vi "Read Photometric Concentration.vi"(8 "error in":errorcluster, 11 "TSI 3022 in":refnum<class "TSI 3022.lvclass">) -> (0 "error out":errorcluster, 2 "Concentration":i32, 3 "TSI 3022 out":refnum<class "TSI 3022.lvclass">)   [LabVIEW 2013, in "TSI 3022.lvclass"]
uses:
  TSI 3022.lvclass
  CPC.lvclass/CPC.ctl
  Accessors/Read Session Handle.vi
  Accessors/Write Session Handle.vi
  Reusable/Session APIs/Serial/Public/Get Data/Get Long Integer.vi
  Reusable/Session APIs/Serial/Serial Session.lvclass
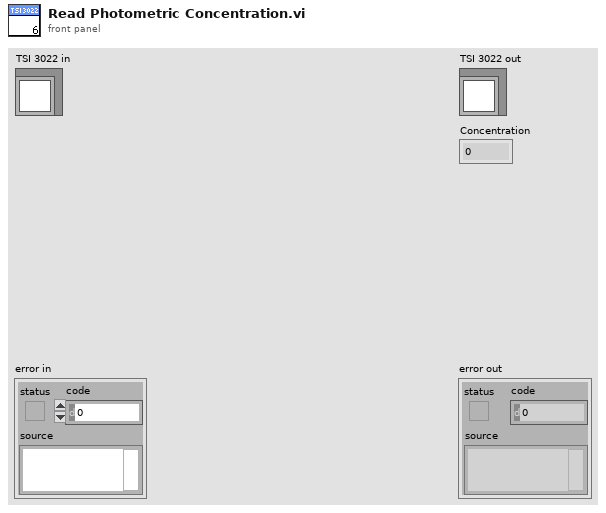
[diagram p1: front panel]
types:
  T1 = typedef "Serial Session.lvclass/Session Handle.ctl" = refnum<data-value>
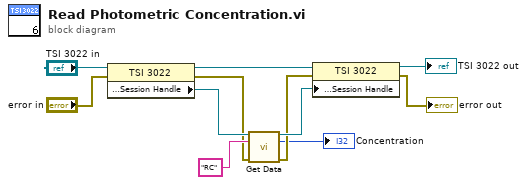
[diagram p0: block diagram]
diagram:
  n1 = property class="TSI 3022"(reference="TSI 3022 in", error in="error in") -> (reference out=w8:refnum<class "TSI 3022.lvclass">, error out=w7:errorcluster, "Accessors:Session Handle"=w10:T1)
  n2 = call-poly "Get Data.vi"("Session Handle in"=w10, "CMD"="RC" ("string"), "error in"=w7) -> ("Session Handle out"=w9:T1, "DataOut"=→"Concentration":i32, "error out"=w6:errorcluster)  [unwired: 10 in]
  n3 = property class="TSI 3022"(reference=w8, error in=w6, "Accessors:Session Handle"=w9) -> (reference out=→"TSI 3022 out":refnum<class "TSI 3022.lvclass">, error out=→"error out":errorcluster)
